vi "SP Append Filter Attenuation Limit Waveform.vi"(4 "Limit Format":T1, 6 "Measured Parameter":T4={"Stimulus Port"=1, "Response Port"=1} {"Stimulus Port" min=1 step=1; "Response Port" min=1 step=1}, 7 "Attribute Name (NI_ChannelName)":string="NI_ChannelName", 8 "error in (no error)":errorcluster, 10 "Results":T3(array[cluster]), 11 "Waveforms in":waveform(dbl)[](array[waveform])) -> (0 "error out":errorcluster, 3 "Waveforms out":waveform(dbl)[](array[waveform]))   [LabVIEW 2011]
uses:
  TypeDefs/SP Parameter.ctl
  TypeDefs/SP Attenuation Type.ctl
  TypeDefs/SP Format.ctl
  TypeDefs/SP Channel Type.ctl
  Channel Test Status Enumeration.ctl
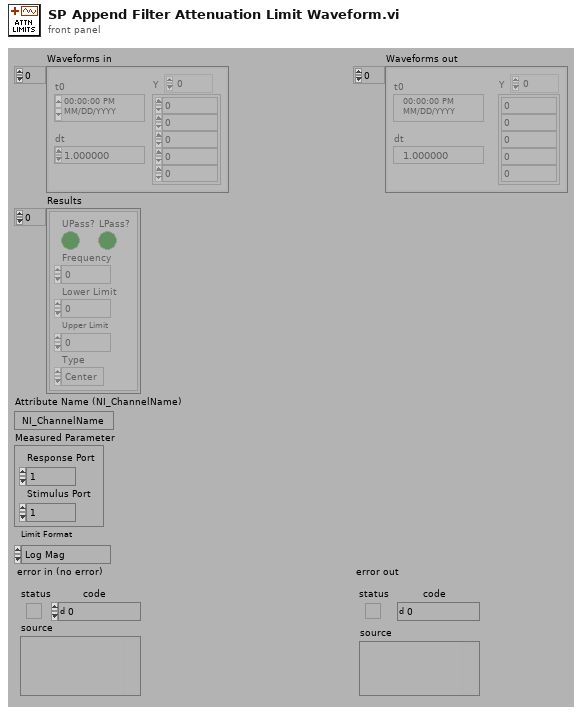
[diagram p1: front panel]
types:
  T1 = typedef "SP Format.ctl" = enum16{"Log Mag", "Lin Mag", "SWR", "Phase", "Expanded Phase", "Delay", "Insertion Loss", "Isolation", "Return Loss"}
  T2 = typedef "SP Attenuation Type.ctl" = enum16{"Center", "Lower", "Upper"}
  T3 = cluster{"UPass?":bool, "LPass?":bool, "Frequency":dbl, "Lower Limit":dbl, "Upper Limit":dbl, "Type":T2}[]
  T4 = typedef "SP Parameter.ctl" = cluster{"Stimulus Port":i8, "Response Port":i8}
  T5 = typedef "SP Channel Type.ctl" = enum16{"Frequency", "Data", "Limit", "Adapter", "Memory", "Value", "Value Limit"}
  T6 = typedef "Channel Test Status Enumeration.ctl" = enum16{"Fail", "Pass", "Abort", "Error", "Done", "Pass by Sample", "Fail by Sample", "Pass Override", "Fail Override", "Not Tested"}
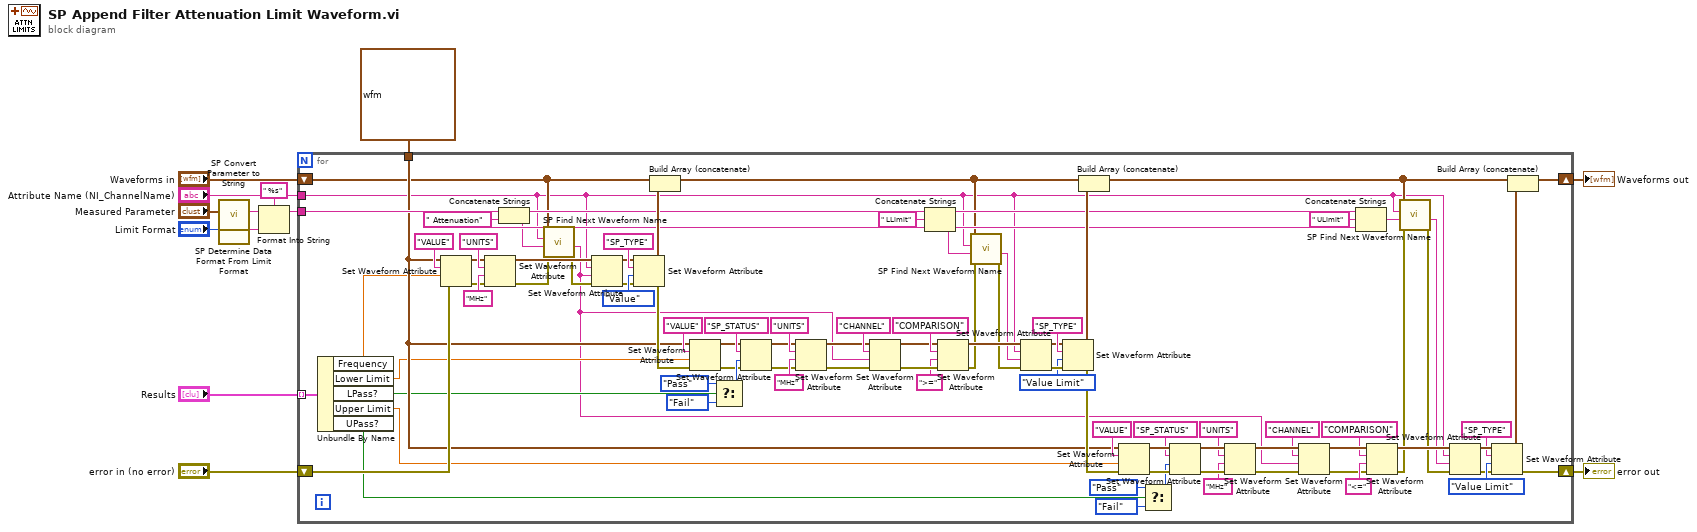
[diagram p0: block diagram]
diagram:
  n1 = call "SP Convert Parameter to String.vi"("Parameter"="Measured Parameter") -> ("Parameter String"=w4:string)  [unwired: 10 out]
  n2 = call "SP Determine Data Format From Limit Format.vi"("Limit Format"="Limit Format") -> ("Format String"=w1:string)
  n3 = Format Into String(format string=" %s", initial string=w4, w1) -> (resulting string=w3:string)  [unwired: 1 in, 1 out]
  n4 = for {
    tunnel: w3 -> [w38]
    tunnel: "Attribute Name (NI_ChannelName)" -> [w14]
    tunnel: waveform(dbl) {"t0"=timestamp(0 s since 1904-01-01), "dt"=1.0, "Y"=[]} ("waveform") -> [w37]
    shift-right: [w40] -> w9
    shift-left: "Waveforms in" -> [w17]
    shift-right: [w42] -> w10
    shift-left: "error in (no error)" -> [w104]
    tunnel: "Results" -> [w36] mode=indexing
    w30 = " Attenuation"
    n5 = Unbundle By Name(w36) -> ("Frequency"=w35:dbl, "Lower Limit"=w33:dbl, "LPass?"=w34:bool, "Upper Limit"=w32:dbl, "UPass?"=w31:bool)
    n6 = Set Waveform Attribute(4:w104, 5:w35, 6:"VALUE", 7:w37) -> (0:w81:errorcluster, 3:w83:waveform(dbl))  [unwired: 1 out]
    n7 = Set Waveform Attribute(4:w81, 5:"MHz", 6:"UNITS", 7:w83) -> (0:w19:errorcluster, 3:w82:waveform(dbl))  [unwired: 1 out]
    n8 = Concatenate Strings(w38, w30) -> (w16:string)
    n9 = call "SP Find Next Waveform Name.vi"("error in (no error)"=w19, "Prospective Base Name"=w16, "Attribute Name (NI_ChannelName)"=w14, "Waveforms in"=w17) -> ("error out"=w18:errorcluster, "Channel Name"=w15:string)  [unwired: 6 in]
    n10 = Set Waveform Attribute(4:w18, 5:w15, 6:w14, 7:w82) -> (0:w91:errorcluster, 3:w92:waveform(dbl))  [unwired: 1 out]
    n11 = Set Waveform Attribute(4:w91, 5:SP_Channel_Type."Value" ("Channel Type"), 6:"SP_TYPE", 7:w92) -> (0:w75:errorcluster, 3:w90:waveform(dbl))  [unwired: 1 out]
    n12 = Build Array (concatenate)(w17, w90) -> (w22:waveform(dbl)[])
    n13 = Set Waveform Attribute(4:w75, 5:w33, 6:"VALUE", 7:w37) -> (0:w74:errorcluster, 3:w73:waveform(dbl))  [unwired: 1 out]
    n14 = Select(t=Channel_Test_Status_Enumeration."Pass" ("Channel Status Enumeration"), s=w34, f=Channel_Test_Status_Enumeration."Fail" ("Channel Status Enumeration")) -> (s? t:f=w100:T6)
    n15 = Set Waveform Attribute(4:w74, 5:w100, 6:"SP_STATUS", 7:w73) -> (0:w84:errorcluster, 3:w85:waveform(dbl))  [unwired: 1 out]
    n16 = Set Waveform Attribute(4:w84, 5:"MHz", 6:"UNITS", 7:w85) -> (0:w79:errorcluster, 3:w78:waveform(dbl))  [unwired: 1 out]
    n17 = Set Waveform Attribute(4:w79, 5:w15, 6:"CHANNEL", 7:w78) -> (0:w69:errorcluster, 3:w71:waveform(dbl))  [unwired: 1 out]
    n18 = Concatenate Strings(w38, " LLimit", w30) -> (w23:string)
    n19 = Set Waveform Attribute(4:w69, 5:">=", 6:"COMPARISON", 7:w71) -> (0:w24:errorcluster, 3:w70:waveform(dbl))  [unwired: 1 out]
    n20 = call "SP Find Next Waveform Name.vi"("error in (no error)"=w24, "Prospective Base Name"=w23, "Attribute Name (NI_ChannelName)"=w14, "Waveforms in"=w22) -> ("error out"=w20:errorcluster, "Channel Name"=w21:string)  [unwired: 6 in]
    n21 = Set Waveform Attribute(4:w20, 5:w21, 6:w14, 7:w70) -> (0:w97:errorcluster, 3:w98:waveform(dbl))  [unwired: 1 out]
    n22 = Set Waveform Attribute(4:w97, 5:SP_Channel_Type."Value Limit" ("Channel Type"), 6:"SP_TYPE", 7:w98) -> (0:w43:errorcluster, 3:w96:waveform(dbl))  [unwired: 1 out]
    n23 = Build Array (concatenate)(w22, w96) -> (w27:waveform(dbl)[])
    n24 = Set Waveform Attribute(4:w43, 5:w32, 6:"VALUE", 7:w37) -> (0:w59:errorcluster, 3:w60:waveform(dbl))  [unwired: 1 out]
    n25 = Select(t=Channel_Test_Status_Enumeration."Pass" ("Channel Status Enumeration"), s=w31, f=Channel_Test_Status_Enumeration."Fail" ("Channel Status Enumeration")) -> (s? t:f=w47:T6)
    n26 = Set Waveform Attribute(4:w59, 5:w47, 6:"SP_STATUS", 7:w60) -> (0:w54:errorcluster, 3:w53:waveform(dbl))  [unwired: 1 out]
    n27 = Set Waveform Attribute(4:w54, 5:"MHz", 6:"UNITS", 7:w53) -> (0:w56:errorcluster, 3:w57:waveform(dbl))  [unwired: 1 out]
    n28 = Set Waveform Attribute(4:w56, 5:w15, 6:"CHANNEL", 7:w57) -> (0:w64:errorcluster, 3:w62:waveform(dbl))  [unwired: 1 out]
    n29 = Concatenate Strings(w38, " ULimit", w30) -> (w29:string)
    n30 = Set Waveform Attribute(4:w64, 5:"<=", 6:"COMPARISON", 7:w62) -> (0:w26:errorcluster, 3:w63:waveform(dbl))  [unwired: 1 out]
    n31 = call "SP Find Next Waveform Name.vi"("error in (no error)"=w26, "Prospective Base Name"=w29, "Attribute Name (NI_ChannelName)"=w14, "Waveforms in"=w27) -> ("error out"=w25:errorcluster, "Channel Name"=w28:string)  [unwired: 6 in]
    n32 = Set Waveform Attribute(4:w25, 5:w28, 6:w14, 7:w63) -> (0:w50:errorcluster, 3:w49:waveform(dbl))  [unwired: 1 out]
    n33 = Set Waveform Attribute(4:w50, 5:SP_Channel_Type."Value Limit" ("Channel Type"), 6:"SP_TYPE", 7:w49) -> (0:w42:errorcluster, 3:w41:waveform(dbl))  [unwired: 1 out]
    n34 = Build Array (concatenate)(w27, w41) -> (w40:waveform(dbl)[])
  }
  "Waveforms out" <- w9
  "error out" <- w10
